vi "FeedForTime.vi"() -> ()   [LabVIEW 2019]
uses:
  Framework/Robot Global Data.vi
panel:
  in  "NoWait?":bool
  in  "Duration":dbl
  in  "Feed":dbl
  in  "Elevate":dbl
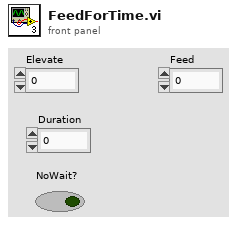
[diagram p1: front panel]
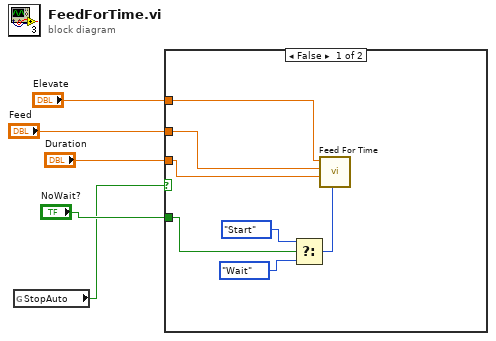
[diagram p0: block diagram]
diagram:
  n1 = global read "Robot Global Data.vi" "StopAuto"() -> (w4:bool)
  n2 = case shown="False" w4 {
    tunnel: "NoWait?" -> [w7 _]
    tunnel: "Elevate" -> [w12 _]
    tunnel: "Feed" -> [w11 _]
    tunnel: "Duration" -> [w10 _]
    frame False {
      n3 = Select(t=enum16{"Start", "Wait"}."Start" ("Synchronization"), s=w7, f=enum16{"Start", "Wait"}."Wait" ("Synchronization")) -> (s? t:f=w6:enum16{"Start", "Wait"})
      n4 = call "Feed For Time.vi"("Lower Setpoint"=w12, "Upper Setpoint"=w11, "Duration (s)"=w10, "Synchronization"=w6) -> ()  [unwired: 6 in, 1 out]
    }
    frame True {
    }
  }
